vi "Global 1.vi"() -> ()   [LabVIEW 2023]
uses:
  Tab_typeDef_lock_state.ctl
panel:
  in  "array_of_clusters_of_all_lockers":T2(array[cluster]) {"lock_state" items=["IDLE", "WORK", "REFILL", "SERVICE", "FAULT"]}
  in  "parcel_placement_time":timestamp
  in  "locations_of_lockers":string[](array[string])
  in  "Location_of_dst_locker_send_glb":string
  in  "Location_of_locker_glb":string
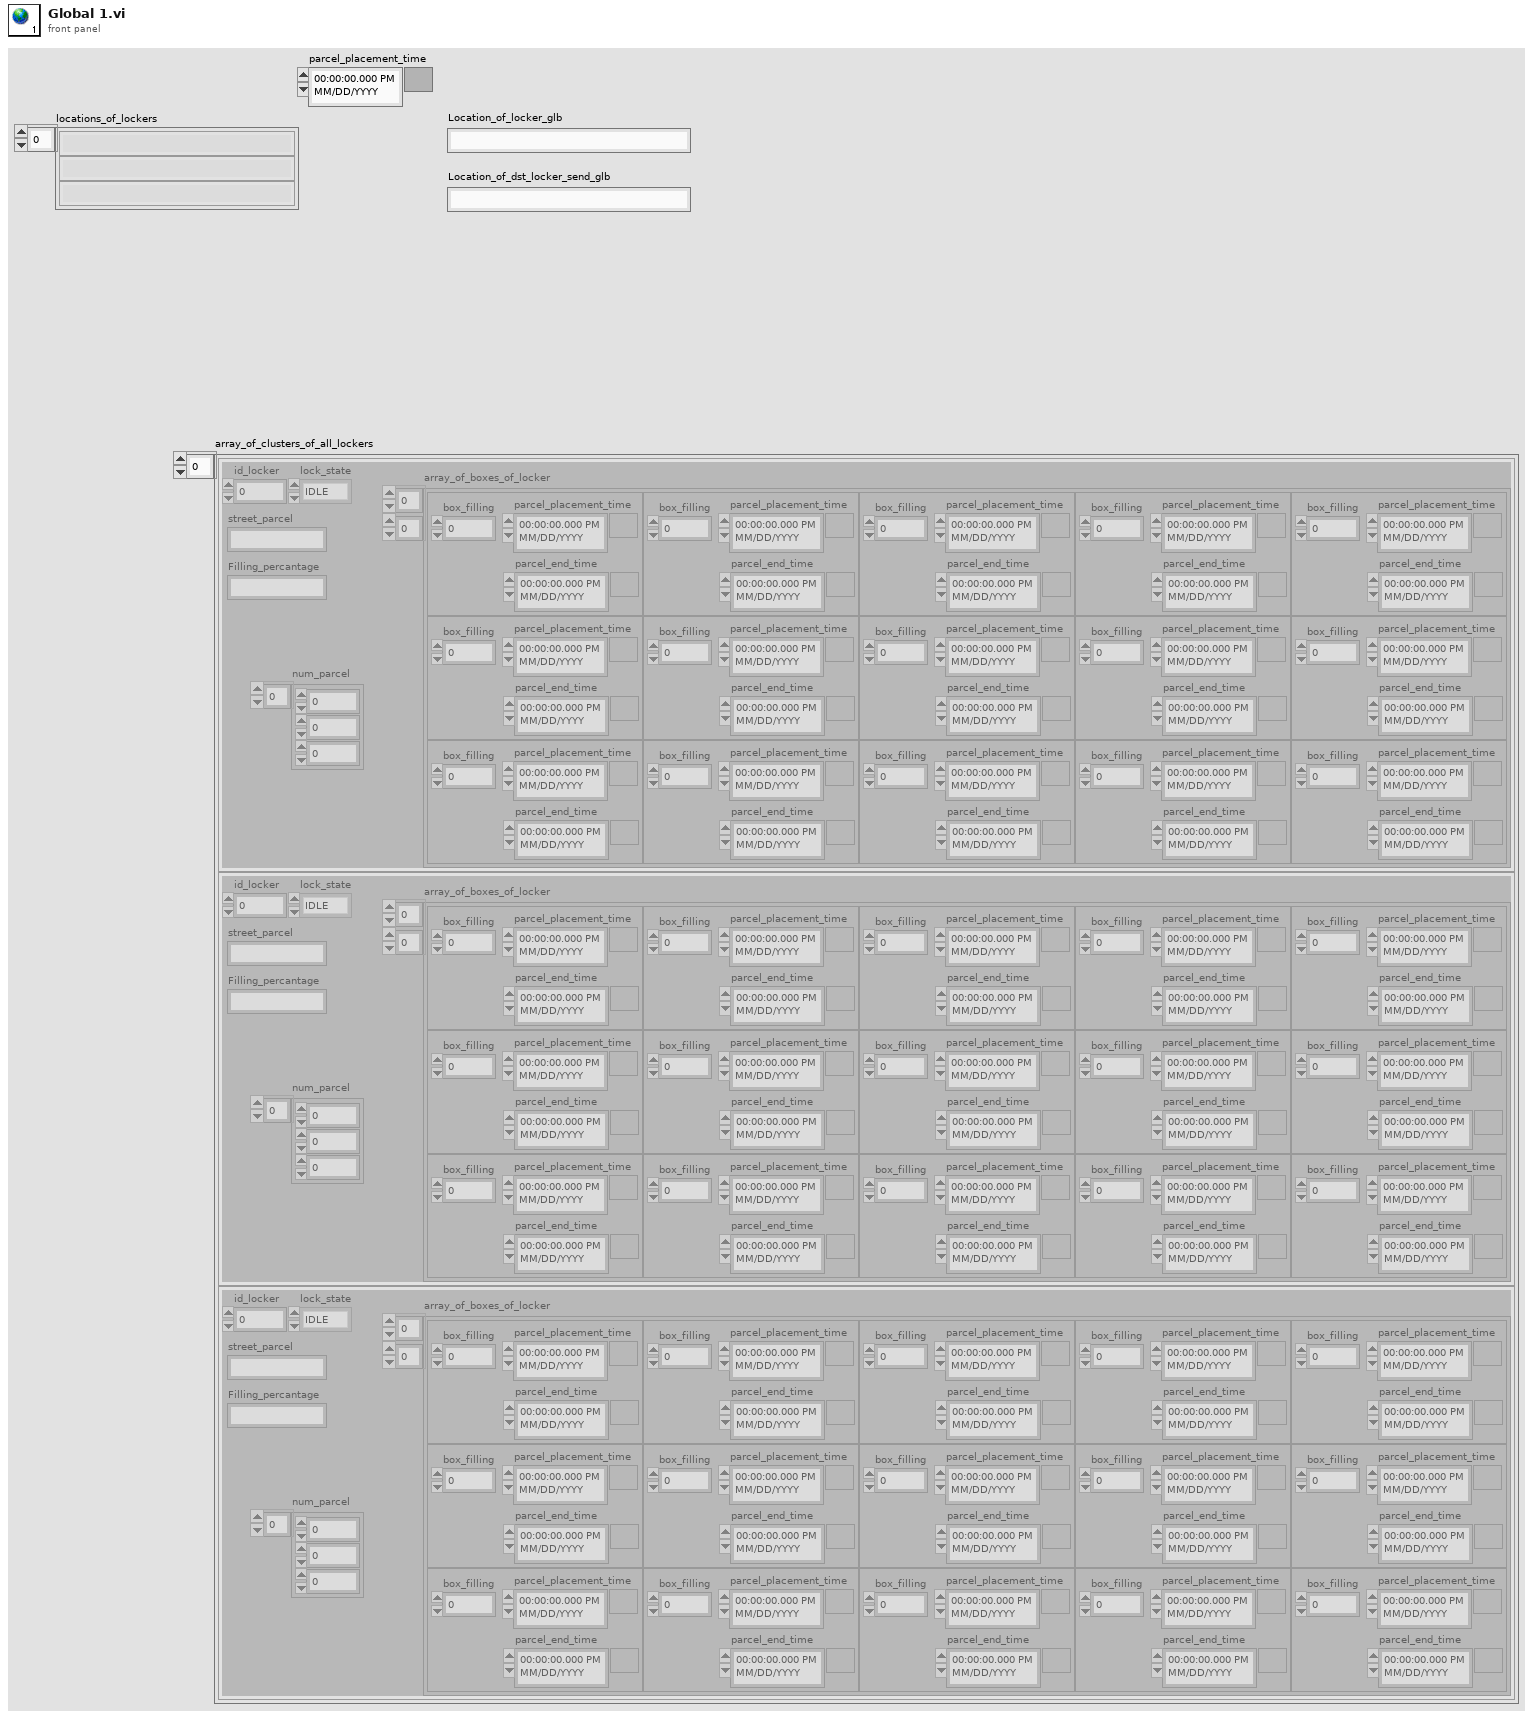
[diagram p1: front panel]
types:
  T1 = typedef "Tab_typeDef_lock_state.ctl" = u16
  T2 = cluster{"id_locker":i32, "street_parcel":string, "lock_state":T1, "Filling_percantage":string, "array_of_boxes_of_locker":cluster{"parcel_end_time":timestamp, "parcel_placement_time":timestamp, "box_filling":dbl}[][], "num_parcel":dbl[]}[]
diagram:
